vi "C4LV_writeFeature.vi"   [LabVIEW 2015, in "libC4HdlLV.lvlib"]
uses:
  libC4HdlLV.lvlib
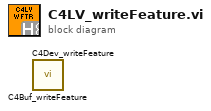
[diagram p0: block diagram]
diagram:
  n1 = call "C4Buf_writeFeature.vi"() -> ()  [unwired: 14 in, 2 out]
  n2 = call "C4Dev_writeFeature.vi"() -> ()  [unwired: 14 in, 2 out]
